vi "Target Colour v2.vi"() -> ()   [LabVIEW 2013]
uses:
  <vilib>/Rock Robotics/WPI/Camera/WPI_CameraSettings Read MJPG.ctl
  <vilib>/Rock Robotics/WPI/Camera/WPI_CameraImageSize.ctl
  <vilib>/vision/NI_Vision_Development_Module.lvlib
panel:
  in  "Camera view angle":dbl=33.7 format="%#_13g"
  out "Distance (cm)":dbl=163.65164688042847
  out "Number of Particles":i32=1
  out "Threshold Image":T1(plugin-control)
  in  "Blue or Luminance":cluster{i32, i32}(slide)={130, 255} scale=0.0..255.0
  in  "Green or Saturation":cluster{i32, i32}(slide)={0, 255} scale=0.0..255.0
  in  "Threshold Color Mode":enum32{"RGB", "HSL"}(radio)=enum."HSL"
  in  "Red or Hue":cluster{i32, i32}(slide)={53, 255} scale=0.0..255.0
  in  "stop":bool
  in  "Camera Settings":T2={"fps"=15, "compression"=5, "Image Size"=enum."320x240"}
  in  "Camera IP":string="10.40.1.11"
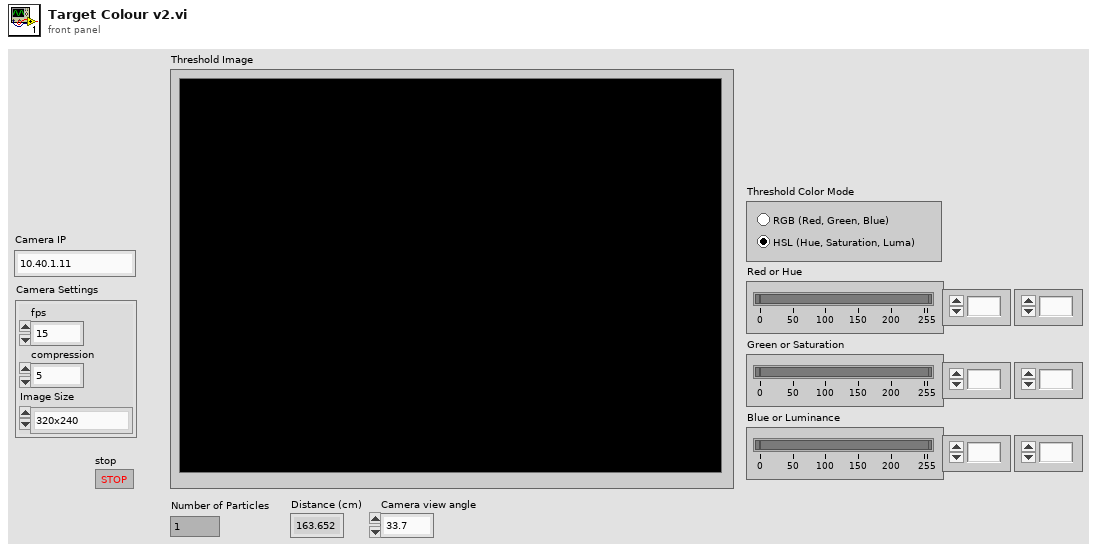
[diagram p1: front panel]
types:
  T1 = typedef "IMAQ Image.ctl" = refnum<image>
  T2 = typedef "WPI_CameraSettings Read MJPG.ctl" = cluster{"fps":i32, "compression":i32, "Image Size":T3}
  T3 = typedef "WPI_CameraImageSize.ctl" = enum16{"640x480", "320x240", "160x120"}
  T4 = typedef "Image Type" = u32
  T5 = typedef "IMAQ Rectangle" = cluster{"Left":i32, "Top":i32, "Right":i32, "Bottom":i32, "Rotation":dbl}
  T6 = typedef "ROI Descriptor" = cluster{"Global Rectangle":i32[], "Contours":cluster{"ID":enum32{"External", "Internal"}, "Type":u32, "Coordinates":i32[]}[]}
  T7 = typedef "Particle Parameters" = i32
  T8 = cluster{"Numeric":dbl, "Numeric":dbl, "Numeric":dbl, "Numeric":dbl}
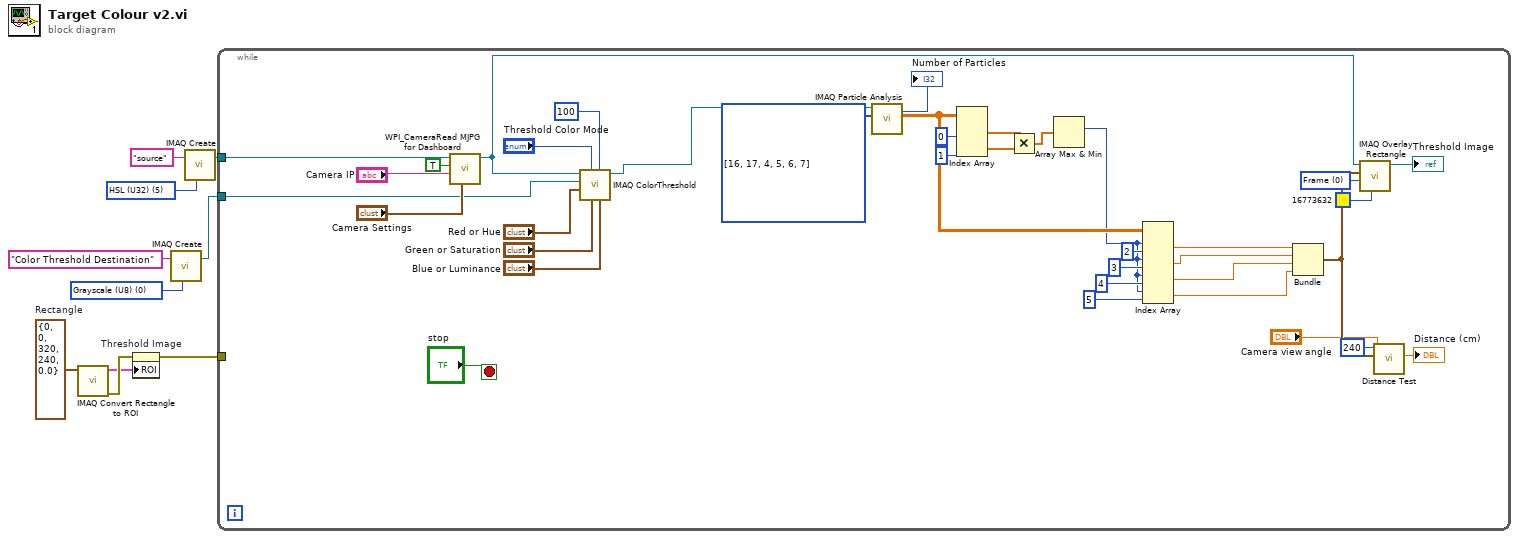
[diagram p0: block diagram]
diagram:
  w4 = T4 0 items=["Grayscale (U8)", "Grayscale (I16)", "Grayscale (SGL)", "Complex (CSG)", "RGB (U32)", "HSL (U32)", "RGB (U64)", "Grayscale (U16)"] ("Image Type")
  w7 = T5 {"Left"=0, "Top"=0, "Right"=320, "Bottom"=240, "Rotation"=0.0}  # Rectangle
  w8 = T4 5 items=["Grayscale (U8)", "Grayscale (I16)", "Grayscale (SGL)", "Complex (CSG)", "RGB (U32)", "HSL (U32)", "RGB (U64)", "Grayscale (U16)"] ("Image Type")
  n1 = call "IMAQ Convert Rectangle to ROI"("Rectangle"=w7) -> ("error out"=w6:errorcluster, "ROI Descriptor"=w5:T6)  [unwired: 8 in]
  n2 = property on="Threshold Image" class="ImageControl"(error in=w6, "ROI"=w5) -> (error out=w1:errorcluster)  [unwired: 1 in, 1 out]
  n3 = call "IMAQ Create"("Image Name"="Color Threshold Destination", "Image Type"=w4) -> ("New Image"=w3:T1)  [unwired: 3 in, 1 out]
  n4 = call "IMAQ Create"("Image Name"="source", "Image Type"=w8) -> ("New Image"=w9:T1)  [unwired: 3 in, 1 out]
  n5 = while {
    tunnel: w9 -> [w43]
    tunnel: w3 -> [w36]
    tunnel: w1 -> [_]
    stop <- "stop" stop-if-true
    w17 = T7[] [16, 17, 4, 5, 6, 7] items=["Center of Mass X", "Center of Mass Y", "First Pixel X", "First Pixel Y", "Bounding Rect Left", "Bounding Rect Top", "Bounding Rect Right", "Bounding Rect Bottom", "Max Feret Diameter Start X", "Max Feret Diameter Start Y", "Max Feret Diameter End X", "Max Feret Diameter End Y", "Max Horiz. Segment Length Left", "Max Horiz. Segment Length Right", "Max Horiz. Segment Length Row", "-", "Bounding Rect Width", "Bounding Rect Height", "Bounding Rect Diagonal", "Perimeter", "Convex Hull Perimeter", "Holes' Perimeter", "Max Feret Diameter", "Equivalent Ellipse Major Axis", "Equivalent Ellipse Minor Axis", "Equivalent Ellipse Minor Axis (Feret)", "Equivalent Rect Long Side", "Equivalent Rect Short Side", "Equivalent Rect Diagonal", "Equivalent Rect Short Side (Feret)", "Average Horiz. Segment Length", "Average Vert. Segment Length", "Hydraulic Radius", "Waddel Disk Diameter", "-", "Area", "Holes' Area", "Particle & Holes' Area", "Convex Hull Area", "Image Area", "-", "Number of Holes", "Number of Horiz. Segments", "Number of Vert. Segments", "-", "Orientation", "Max Feret Diameter Orientation", "-", "% Area/Image Area", "% Area/(Particle & Holes' Area)", "Ratio of Equivalent Ellipse Axes", "Ratio of Equivalent Rect Sides", "-", "Elongation Factor", "Compactness Factor", "Heywood Circularity Factor", "Type Factor", "-", "Sum X", "Sum Y", "Sum XX", "Sum XY", "Sum YY", "Sum XXX", "Sum XXY", "Sum XYY", "Sum YYY", "-", "Moment of Inertia XX", "Moment of Inertia XY", "Moment of Inertia YY", "Moment of Inertia XXX", "Moment of Inertia XXY", "Moment of Inertia XYY", "Moment of Inertia YYY", "Norm. Moment of Inertia XX", "Norm. Moment of Inertia XY", "Norm. Moment of Inertia YY", "Norm. Moment of Inertia XXX", "Norm. Moment of Inertia XXY", "Norm. Moment of Inertia XYY", "Norm. Moment of Inertia YYY", "Hu Moment 1", "Hu Moment 2", "Hu Moment 3", "Hu Moment 4", "Hu Moment 5", "Hu Moment 6", "Hu Moment 7"] ("Pixel Measurements")
    w41 = u32 0 items=["Frame", "Fill", "Highlight"] ("Drawing Mode (Frame)")
    n6 = call <vilib>:"WPI_CameraRead MJPG for Dashboard.vi"("Camera Settings"="Camera Settings", "Camera IP"="Camera IP", "Enable"=TRUE, "Refnum in"=w43) -> ("Refnum out"=w11:T1)  [unwired: 4 in, 3 out]
    n7 = call "IMAQ ColorThreshold"("Blue or Luma or Val or Inten Range"="Blue or Luminance", "Replace Value"=100, "Green or Sat Range"="Green or Saturation", "Color Mode"="Threshold Color Mode", "Red or Hue Range"="Red or Hue", "Image Dst"=w36, "Image Src"=w11) -> ("Image Dst Out"=w16:T1)  [unwired: 3 in, 1 out]
    n8 = call "IMAQ Particle Analysis"("Pixel Measurements"=w17, "Image"=w16) -> ("Particle Measurements (Pixels)"=w29:dbl[][], "Number of Particles"=→"Number of Particles":i32)  [unwired: 3 in, 5 out]
    n9 = Index Array(array=w29, index (col) #1=0 ("disabled index (col)"), index (col) #2=1 ("index (col)")) -> (element #1=w32:dbl[], element #2=w31:dbl[])  [unwired: 2 in]
    n10 = Multiply(x=w32, y=w31) -> (x*y=w30:dbl[])
    n11 = Array Max & Min(array=w30) -> (max index (indices)=w20:i32)  [unwired: 3 out]
    n12 = Index Array(array=w29, index (row) #1=w20, index (col) #1=2 ("disabled index (col)"), index (row) #2=w20, index (col) #2=3 ("index (col)"), index (row) #3=w20, index (col) #3=4 ("index (col)"), index (row) #4=w20, index (col) #4=5 ("index (col)")) -> (element #1=w26:dbl, element #2=w25:dbl, element #3=w22:dbl, element #4=w21:dbl)
    n13 = Bundle("Numeric"=w26, "Numeric"=w25, "Numeric"=w22, "Numeric"=w21) -> (w15:T8)  [unwired: 1 in]
    n14 = call "IMAQ Overlay Rectangle"("Color"=u32 16773632, "Drawing Mode (Frame)"=w41, "Rectangle"=w15, "Image"=w11) -> ("Image Out"=→"Threshold Image":T1)  [unwired: 6 in, 1 out]
    n15 = call "Distance Test.vi"("Camera view angle"="Camera view angle", "Rectangle"=w15, "Y Image Resolution"=240) -> ("Distance (cm)"=→"Distance (cm)":dbl)  [unwired: 8 in]
  }
